vi "15T_Merge_Cluster.vi"(1 "15T-Status":T1, 3 "15T-Control":T2={"Setpoint (T)"=3.4572, "Rate (T/min)"=0.0, "Go to zero"=FALSE, "Go to Hold"=FALSE, "Go to Set"=FALSE, "Clamp"=FALSE, "Switch Heater"=FALSE} {"Rate (T/min)" format="%6_5f"; "Setpoint (T)" format="%6_5f"}) -> (0 "15T-Cluster":T3={"Magnet (T)"=0.0, "Leads (T)"=0.0, "Setpoint (T)"=3.4572, "Rate (T/min)"=0.0, "Set"=FALSE, "Zero"=FALSE, "Hold"=FALSE, "Go to zero"=FALSE, "Go to Hold"=FALSE, "Go to Set"=FALSE, "Clamp"=FALSE, "Switch Heater"=FALSE, "Rate limit"=FALSE, "Switch"=FALSE, "Clamped"=FALSE, "Persistent"=FALSE, "Quenched"=FALSE, "Sweeping"=FALSE, "Select"=FALSE} {"Rate (T/min)" format="%6_5f"; "Setpoint (T)" format="%6_5f"})   [LabVIEW 2019]
uses:
  Berta/15T-Cluster.ctl
  Berta/15T-Control.ctl
  Berta/15T-Status.ctl
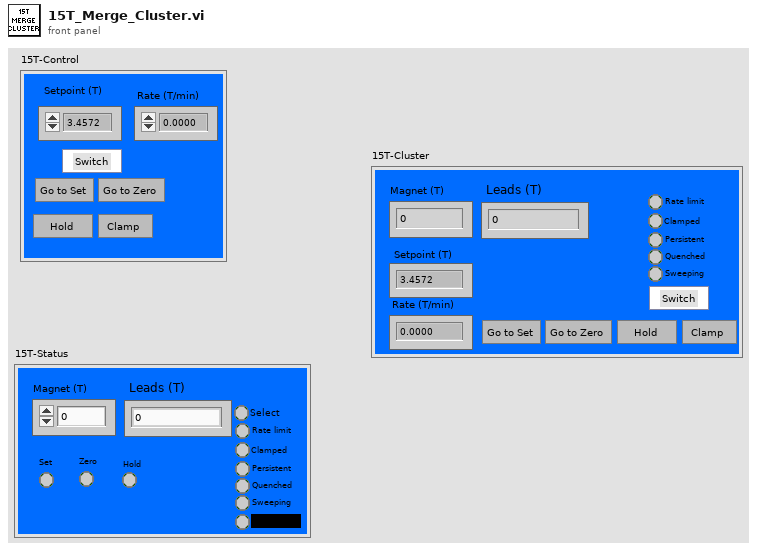
[diagram p1: front panel]
types:
  T1 = typedef "15T-Status.ctl" = cluster{"Magnet (T)":dbl, "Leads (T)":dbl, "Set":bool, "Zero":bool, "Hold":bool, "Rate limit":bool, "Switch":bool, "Clamped":bool, "Persistent":bool, "Quenched":bool, "Sweeping":bool, "Select":bool}
  T2 = typedef "15T-Control.ctl" = cluster{"Setpoint (T)":dbl, "Rate (T/min)":dbl, "Go to zero":bool, "Go to Hold":bool, "Go to Set":bool, "Clamp":bool, "Switch Heater":bool}
  T3 = typedef "15T-Cluster.ctl" = cluster{"Magnet (T)":dbl, "Leads (T)":dbl, "Setpoint (T)":dbl, "Rate (T/min)":dbl, "Set":bool, "Zero":bool, "Hold":bool, "Go to zero":bool, "Go to Hold":bool, "Go to Set":bool, "Clamp":bool, "Switch Heater":bool, "Rate limit":bool, "Switch":bool, "Clamped":bool, "Persistent":bool, "Quenched":bool, "Sweeping":bool, "Select":bool}
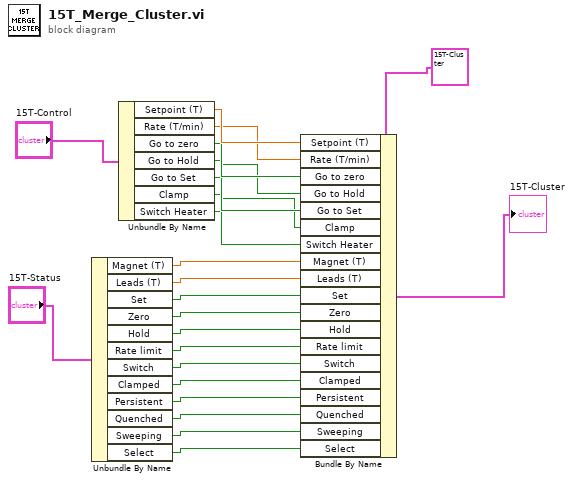
[diagram p0: block diagram]
diagram:
  n1 = Unbundle By Name("15T-Status") -> ("Magnet (T)"=w12:dbl, "Leads (T)"=w11:dbl, "Set"=w10:bool, "Zero"=w9:bool, "Hold"=w8:bool, "Rate limit"=w7:bool, "Switch"=w6:bool, "Clamped"=w5:bool, "Persistent"=w4:bool, "Quenched"=w3:bool, "Sweeping"=w2:bool, "Select"=w1:bool)
  n2 = Unbundle By Name("15T-Control") -> ("Setpoint (T)"=w19:dbl, "Rate (T/min)"=w18:dbl, "Go to zero"=w17:bool, "Go to Hold"=w16:bool, "Go to Set"=w15:bool, "Clamp"=w14:bool, "Switch Heater"=w13:bool)
  n3 = Bundle By Name(cluster=T3 {"Magnet (T)"=0.0, "Leads (T)"=0.0, "Setpoint (T)"=3.4572, "Rate (T/min)"=0.0, "Set"=FALSE, "Zero"=FALSE, "Hold"=FALSE, "Go to zero"=FALSE, "Go to Hold"=FALSE, "Go to Set"=FALSE, "Clamp"=FALSE, "Switch Heater"=FALSE, "Rate limit"=FALSE, "Switch"=FALSE, "Clamped"=FALSE, "Persistent"=FALSE, "Quenched"=FALSE, "Sweeping"=FALSE, "Select"=FALSE} ("15T-Cluster"), "Setpoint (T)"=w19, "Rate (T/min)"=w18, "Go to zero"=w17, "Go to Hold"=w16, "Go to Set"=w15, "Clamp"=w14, "Switch Heater"=w13, "Magnet (T)"=w12, "Leads (T)"=w11, "Set"=w10, "Zero"=w9, "Hold"=w8, "Rate limit"=w7, "Switch"=w6, "Clamped"=w5, "Persistent"=w4, "Quenched"=w3, "Sweeping"=w2, "Select"=w1) -> (→"15T-Cluster":T3)
